vi "TemperatureMeasureDT.vi"(1 "FieldPoint IO Point In":refnum<k21>) -> (0 "Ch2 [K]":dbl)   [LabVIEW 2012]
uses:
  <vilib>/FieldPoint/Polymorphic Read.llb/FP Read (Float -IO).vi
panel:
  in  "?":bool
  # "Temperature Measurement (DT 670)"
  # "(Recommended excitation 10 µA  ±0.1%)"
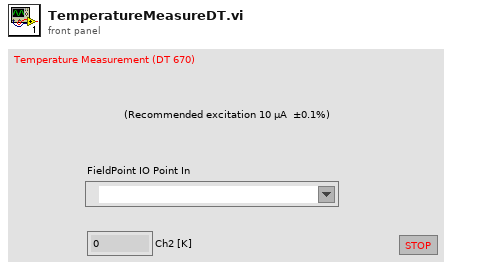
[diagram p1: front panel]
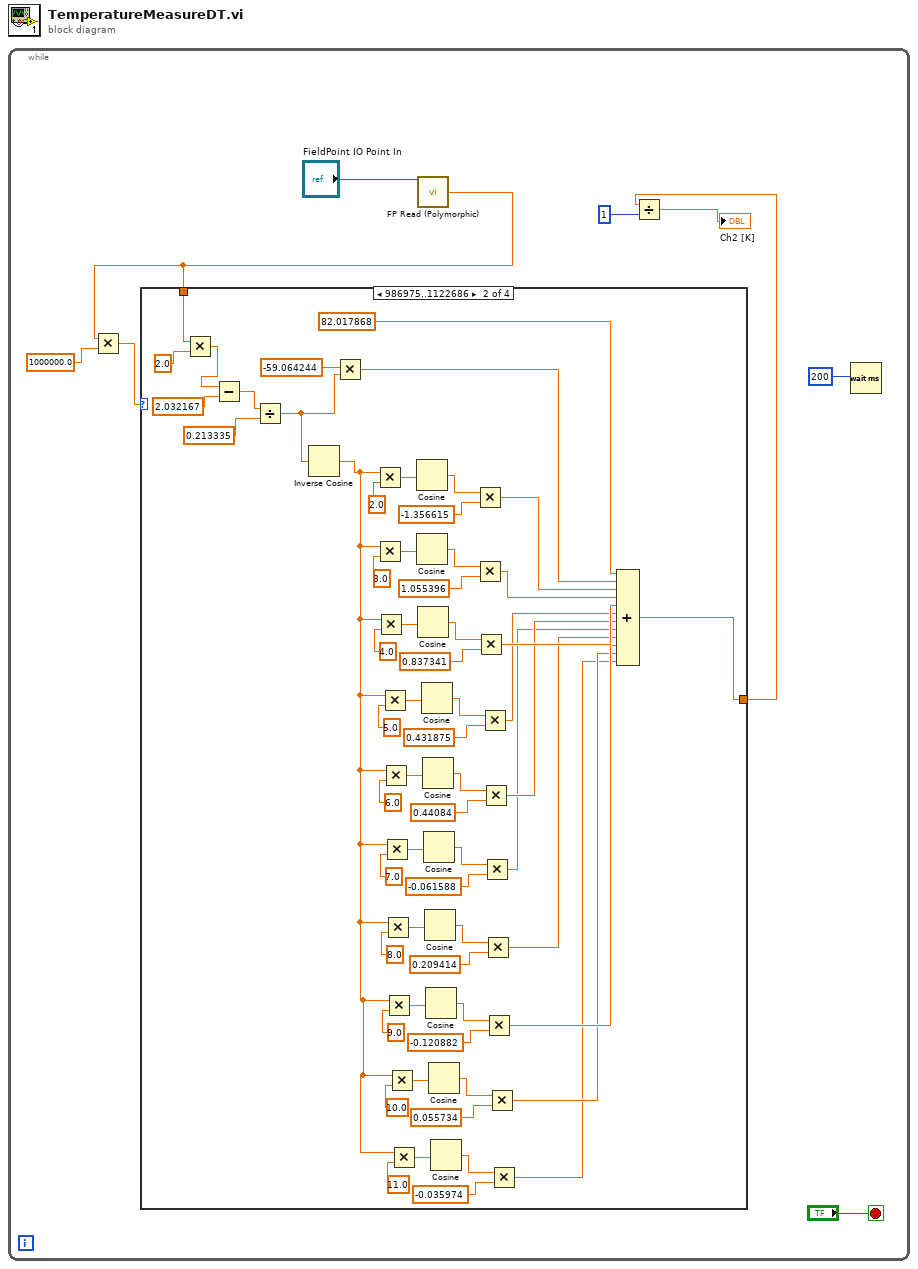
[diagram p0: block diagram]
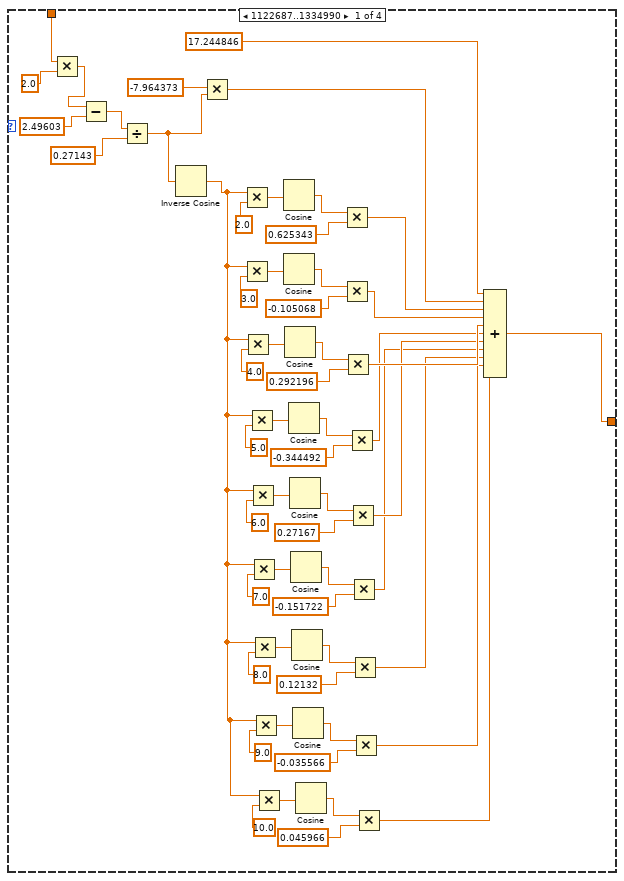
[diagram p2: hidden frame]
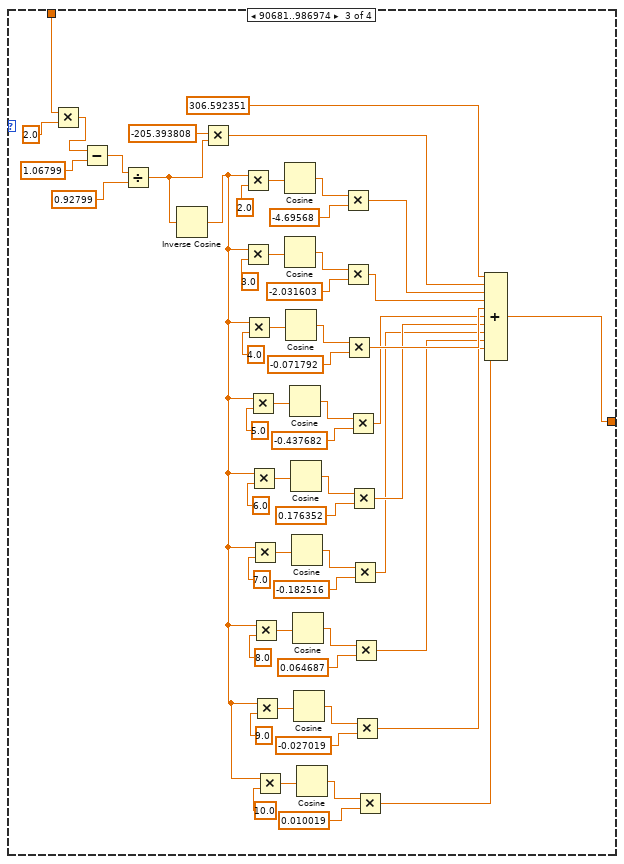
[diagram p3: hidden frame]
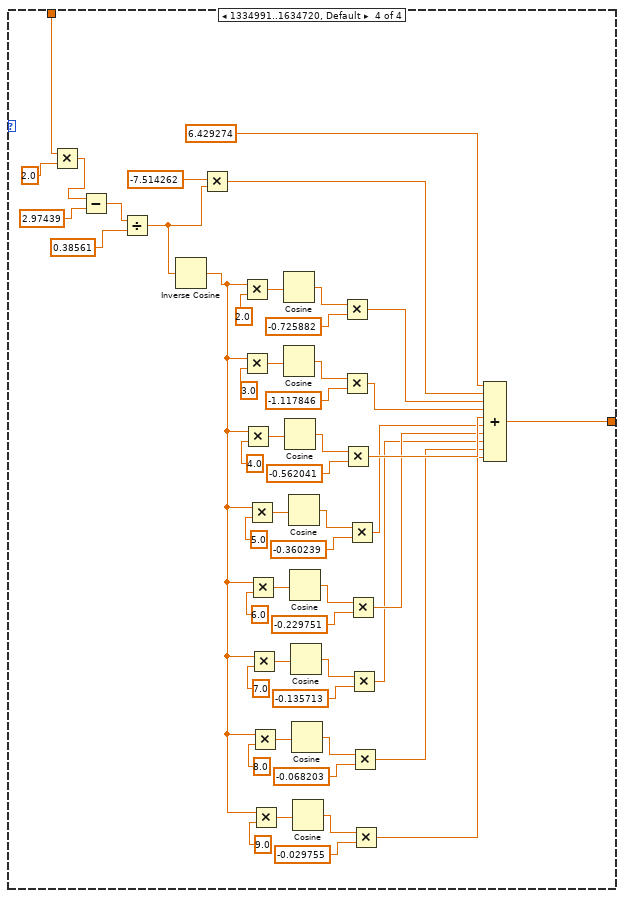
[diagram p4: hidden frame]
diagram:
  n1 = while {
    stop <- "?" stop-if-true
    n2 = call-poly <vilib>:"FP Read (Polymorphic).vi"("FieldPoint IO Point In"="FieldPoint IO Point In") -> ("value"=w4:dbl)  [unwired: 11 in, 3 out]
    n3 = Multiply(x=w4, y=1000000.0) -> (x*y=w5:dbl)
    n4 = case shown="986975..1122686" w5 {
      tunnel: w4 -> [w17 w74 w130 w236]
      tunnel: [w10 w73 w129 w186] -> w2
      frame 1122687..1334990 {
        n5 = Multiply(x=w17, y=2.0) -> (x*y=w65:dbl)
        n6 = Subtract(x=w65, y=2.49603) -> (x-y=w63:dbl)
        n7 = Divide(x=w63, y=0.27143) -> (x/y=w60:dbl)
        n8 = Inverse Cosine(1:w60) -> (0:w12:dbl)
        n9 = Multiply(x=-7.964373, y=w60) -> (x*y=w26:dbl)
        n10 = Multiply(x=w12, y=2.0) -> (x*y=w58:dbl)
        n11 = Multiply(x=w12, y=3.0) -> (x*y=w54:dbl)
        n12 = Multiply(x=w12, y=4.0) -> (x*y=w50:dbl)
        n13 = Multiply(x=w12, y=5.0) -> (x*y=w46:dbl)
        n14 = Multiply(x=w12, y=6.0) -> (x*y=w42:dbl)
        n15 = Multiply(x=w12, y=7.0) -> (x*y=w38:dbl)
        n16 = Multiply(x=w12, y=8.0) -> (x*y=w34:dbl)
        n17 = Multiply(x=w12, y=9.0) -> (x*y=w30:dbl)
        n18 = Multiply(x=w12, y=10.0) -> (x*y=w15:dbl)
        n19 = Cosine(x=w58) -> (cos(x)=w57:dbl)
        n20 = Cosine(x=w54) -> (cos(x)=w53:dbl)
        n21 = Cosine(x=w50) -> (cos(x)=w49:dbl)
        n22 = Cosine(x=w46) -> (cos(x)=w45:dbl)
        n23 = Cosine(x=w42) -> (cos(x)=w41:dbl)
        n24 = Cosine(x=w38) -> (cos(x)=w37:dbl)
        n25 = Cosine(x=w34) -> (cos(x)=w33:dbl)
        n26 = Cosine(x=w30) -> (cos(x)=w29:dbl)
        n27 = Cosine(x=w15) -> (cos(x)=w14:dbl)
        n28 = Multiply(x=w57, y=0.625343) -> (x*y=w25:dbl)
        n29 = Multiply(x=w53, y=-0.105068) -> (x*y=w24:dbl)
        n30 = Multiply(x=w49, y=0.292196) -> (x*y=w23:dbl)
        n31 = Multiply(x=w45, y=-0.344492) -> (x*y=w22:dbl)
        n32 = Multiply(x=w41, y=0.27167) -> (x*y=w21:dbl)
        n33 = Multiply(x=w37, y=-0.151722) -> (x*y=w20:dbl)
        n34 = Multiply(x=w33, y=0.12132) -> (x*y=w19:dbl)
        n35 = Multiply(x=w29, y=-0.035566) -> (x*y=w18:dbl)
        n36 = Multiply(x=w14, y=0.045966) -> (x*y=w11:dbl)
        n37 = Compound Arithmetic op=ADD(17.244846, w26, w25, w24, w23, w22, w21, w20, w19, w18, w11) -> (w10:dbl)
      }
      frame 986975..1122686 {
        n38 = Multiply(x=w74, y=2.0) -> (x*y=w127:dbl)
        n39 = Subtract(x=w127, y=2.032167) -> (x-y=w125:dbl)
        n40 = Divide(x=w125, y=0.213335) -> (x/y=w122:dbl)
        n41 = Inverse Cosine(1:w122) -> (0:w68:dbl)
        n42 = Multiply(x=-59.064244, y=w122) -> (x*y=w88:dbl)
        n43 = Multiply(x=w68, y=2.0) -> (x*y=w120:dbl)
        n44 = Multiply(x=w68, y=3.0) -> (x*y=w116:dbl)
        n45 = Multiply(x=w68, y=4.0) -> (x*y=w112:dbl)
        n46 = Multiply(x=w68, y=5.0) -> (x*y=w108:dbl)
        n47 = Multiply(x=w68, y=6.0) -> (x*y=w104:dbl)
        n48 = Multiply(x=w68, y=7.0) -> (x*y=w100:dbl)
        n49 = Multiply(x=w68, y=8.0) -> (x*y=w96:dbl)
        n50 = Multiply(x=w68, y=9.0) -> (x*y=w92:dbl)
        n51 = Multiply(x=w68, y=10.0) -> (x*y=w78:dbl)
        n52 = Multiply(x=w68, y=11.0) -> (x*y=w71:dbl)
        n53 = Cosine(x=w120) -> (cos(x)=w119:dbl)
        n54 = Cosine(x=w116) -> (cos(x)=w115:dbl)
        n55 = Cosine(x=w112) -> (cos(x)=w111:dbl)
        n56 = Cosine(x=w108) -> (cos(x)=w107:dbl)
        n57 = Cosine(x=w104) -> (cos(x)=w103:dbl)
        n58 = Cosine(x=w100) -> (cos(x)=w99:dbl)
        n59 = Cosine(x=w96) -> (cos(x)=w95:dbl)
        n60 = Cosine(x=w92) -> (cos(x)=w91:dbl)
        n61 = Cosine(x=w78) -> (cos(x)=w77:dbl)
        n62 = Cosine(x=w71) -> (cos(x)=w70:dbl)
        n63 = Multiply(x=w119, y=-1.356615) -> (x*y=w87:dbl)
        n64 = Multiply(x=w115, y=1.055396) -> (x*y=w86:dbl)
        n65 = Multiply(x=w111, y=0.837341) -> (x*y=w85:dbl)
        n66 = Multiply(x=w107, y=0.431875) -> (x*y=w84:dbl)
        n67 = Multiply(x=w103, y=0.44084) -> (x*y=w83:dbl)
        n68 = Multiply(x=w99, y=-0.061588) -> (x*y=w82:dbl)
        n69 = Multiply(x=w95, y=0.209414) -> (x*y=w81:dbl)
        n70 = Multiply(x=w91, y=-0.120882) -> (x*y=w80:dbl)
        n71 = Multiply(x=w77, y=0.055734) -> (x*y=w75:dbl)
        n72 = Multiply(x=w70, y=-0.035974) -> (x*y=w67:dbl)
        n73 = Compound Arithmetic op=ADD(82.017868, w88, w87, w86, w85, w84, w83, w82, w81, w80, w75, w67) -> (w73:dbl)
      }
      frame 90681..986974 {
        n74 = Multiply(x=w130, y=2.0) -> (x*y=w184:dbl)
        n75 = Subtract(x=w184, y=1.06799) -> (x-y=w182:dbl)
        n76 = Divide(x=w182, y=0.92799) -> (x/y=w179:dbl)
        n77 = Inverse Cosine(1:w179) -> (0:w132:dbl)
        n78 = Multiply(x=-205.393808, y=w179) -> (x*y=w145:dbl)
        n79 = Multiply(x=w132, y=2.0) -> (x*y=w177:dbl)
        n80 = Multiply(x=w132, y=3.0) -> (x*y=w173:dbl)
        n81 = Multiply(x=w132, y=4.0) -> (x*y=w169:dbl)
        n82 = Multiply(x=w132, y=5.0) -> (x*y=w165:dbl)
        n83 = Multiply(x=w132, y=6.0) -> (x*y=w161:dbl)
        n84 = Multiply(x=w132, y=7.0) -> (x*y=w157:dbl)
        n85 = Multiply(x=w132, y=8.0) -> (x*y=w153:dbl)
        n86 = Multiply(x=w132, y=9.0) -> (x*y=w149:dbl)
        n87 = Multiply(x=w132, y=10.0) -> (x*y=w135:dbl)
        n88 = Cosine(x=w177) -> (cos(x)=w176:dbl)
        n89 = Cosine(x=w173) -> (cos(x)=w172:dbl)
        n90 = Cosine(x=w169) -> (cos(x)=w168:dbl)
        n91 = Cosine(x=w165) -> (cos(x)=w164:dbl)
        n92 = Cosine(x=w161) -> (cos(x)=w160:dbl)
        n93 = Cosine(x=w157) -> (cos(x)=w156:dbl)
        n94 = Cosine(x=w153) -> (cos(x)=w152:dbl)
        n95 = Cosine(x=w149) -> (cos(x)=w148:dbl)
        n96 = Cosine(x=w135) -> (cos(x)=w134:dbl)
        n97 = Multiply(x=w176, y=-4.69568) -> (x*y=w144:dbl)
        n98 = Multiply(x=w172, y=-2.031603) -> (x*y=w143:dbl)
        n99 = Multiply(x=w168, y=-0.071792) -> (x*y=w142:dbl)
        n100 = Multiply(x=w164, y=-0.437682) -> (x*y=w141:dbl)
        n101 = Multiply(x=w160, y=0.176352) -> (x*y=w140:dbl)
        n102 = Multiply(x=w156, y=-0.182516) -> (x*y=w139:dbl)
        n103 = Multiply(x=w152, y=0.064687) -> (x*y=w138:dbl)
        n104 = Multiply(x=w148, y=-0.027019) -> (x*y=w137:dbl)
        n105 = Multiply(x=w134, y=0.010019) -> (x*y=w131:dbl)
        n106 = Compound Arithmetic op=ADD(306.592351, w145, w144, w143, w142, w141, w140, w139, w138, w137, w131) -> (w129:dbl)
      }
      frame 1334991..1634720, Default {
        n107 = Multiply(x=w236, y=2.0) -> (x*y=w235:dbl)
        n108 = Subtract(x=w235, y=2.97439) -> (x-y=w233:dbl)
        n109 = Divide(x=w233, y=0.38561) -> (x/y=w230:dbl)
        n110 = Inverse Cosine(1:w230) -> (0:w197:dbl)
        n111 = Multiply(x=-7.514262, y=w230) -> (x*y=w195:dbl)
        n112 = Multiply(x=w197, y=2.0) -> (x*y=w228:dbl)
        n113 = Multiply(x=w197, y=3.0) -> (x*y=w224:dbl)
        n114 = Multiply(x=w197, y=4.0) -> (x*y=w220:dbl)
        n115 = Multiply(x=w197, y=5.0) -> (x*y=w216:dbl)
        n116 = Multiply(x=w197, y=6.0) -> (x*y=w212:dbl)
        n117 = Multiply(x=w197, y=7.0) -> (x*y=w208:dbl)
        n118 = Multiply(x=w197, y=8.0) -> (x*y=w204:dbl)
        n119 = Multiply(x=w197, y=9.0) -> (x*y=w200:dbl)
        n120 = Cosine(x=w228) -> (cos(x)=w227:dbl)
        n121 = Cosine(x=w224) -> (cos(x)=w223:dbl)
        n122 = Cosine(x=w220) -> (cos(x)=w219:dbl)
        n123 = Cosine(x=w216) -> (cos(x)=w215:dbl)
        n124 = Cosine(x=w212) -> (cos(x)=w211:dbl)
        n125 = Cosine(x=w208) -> (cos(x)=w207:dbl)
        n126 = Cosine(x=w204) -> (cos(x)=w203:dbl)
        n127 = Cosine(x=w200) -> (cos(x)=w199:dbl)
        n128 = Multiply(x=w227, y=-0.725882) -> (x*y=w194:dbl)
        n129 = Multiply(x=w223, y=-1.117846) -> (x*y=w193:dbl)
        n130 = Multiply(x=w219, y=-0.562041) -> (x*y=w192:dbl)
        n131 = Multiply(x=w215, y=-0.360239) -> (x*y=w191:dbl)
        n132 = Multiply(x=w211, y=-0.229751) -> (x*y=w190:dbl)
        n133 = Multiply(x=w207, y=-0.135713) -> (x*y=w189:dbl)
        n134 = Multiply(x=w203, y=-0.068203) -> (x*y=w188:dbl)
        n135 = Multiply(x=w199, y=-0.029755) -> (x*y=w187:dbl)
        n136 = Compound Arithmetic op=ADD(6.429274, w195, w194, w193, w192, w191, w190, w189, w188, w187) -> (w186:dbl)
      }
    }
    n137 = Divide(x=w2, y=1) -> (x/y=→"Ch2 [K]":dbl)
    n138 = Wait (ms)(milliseconds to wait=u32 200) -> ()  [unwired: 1 out]
  }
